vi "uTTA_CheckForErrors.vi"(8 "error in":errorcluster, 11 "Received":string) -> (0 "error out":errorcluster)   [LabVIEW 2021]
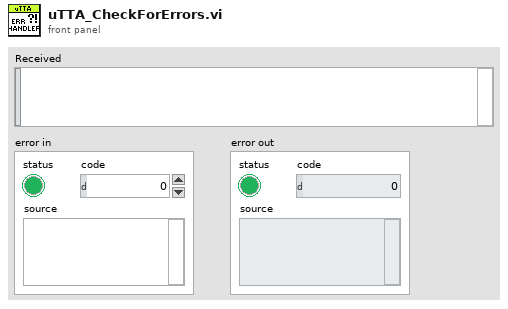
[diagram p1: front panel]
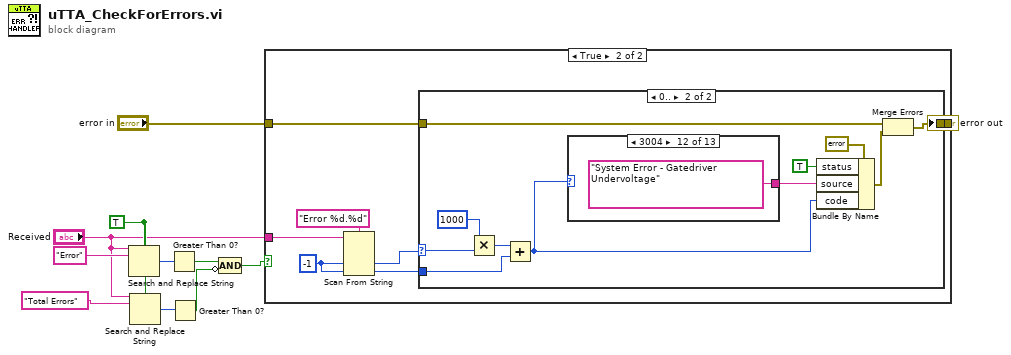
[diagram p0: block diagram]
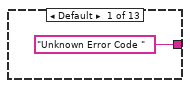
[diagram p4: hidden frame]
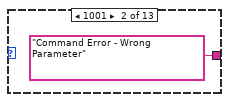
[diagram p5: hidden frame]
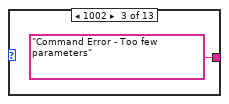
[diagram p6: hidden frame]
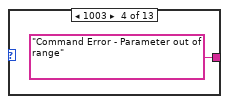
[diagram p7: hidden frame]
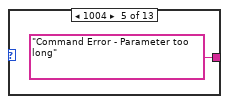
[diagram p8: hidden frame]
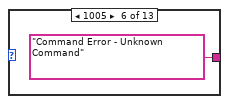
[diagram p9: hidden frame]
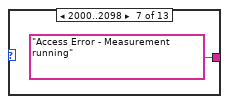
[diagram p10: hidden frame]
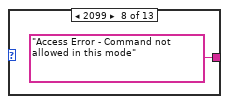
[diagram p11: hidden frame]
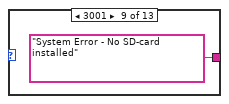
[diagram p12: hidden frame]
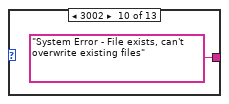
[diagram p13: hidden frame]
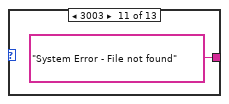
[diagram p14: hidden frame]
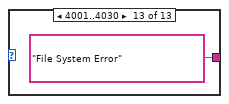
[diagram p15: hidden frame]
diagram:
  w8 = TRUE ("ignore case? (F)")
  n1 = Search and Replace String(case sensitive?=w8, input string="Received", search string="Error" ("format string")) -> (number of replacements=w4:i32)  [unwired: 5 in, 3 out]
  n2 = Search and Replace String(case sensitive?=w8, input string="Received", search string="Total Errors" ("format string")) -> (number of replacements=w5:i32)  [unwired: 5 in, 3 out]
  n3 = Greater Than 0?(x=w4) -> (x > 0?=w3:bool)
  n4 = Greater Than 0?(x=w5) -> (x > 0?=w2:bool)
  n5 = Compound Arithmetic op=AND(w3, invert w2) -> (w1:bool)
  n6 = case shown="True" w1 {
    tunnel: [w12 w19] -> w11
    tunnel: "error in" -> [w12 w18]
    tunnel: "Received" -> [_ w13]
    frame False {
    }
    frame True {
      w16 = -1 ("default value 1")
      n7 = Scan From String(format string="Error %d.%d", input string=w13, default 1=w16, default 2=w16) -> (output 1=w15:i32, output 2=w14:i32)  [unwired: 2 in, 3 out]
      n8 = case shown="0.." w15 {
        selector: w15 -> [_ w23]
        tunnel: w18 -> [w20 w31]
        tunnel: [w20 w30] -> w19
        tunnel: w14 -> [_ w25]
        frame Default {
        }
        frame 0.. {
          n9 = Multiply(x=1000, y=w23) -> (x*y=w22:i32)
          n10 = Add(x=w22, y=w25) -> (x+y=w21:i32)
          n11 = case shown="3004" w21 {
            tunnel: ["Unknown Error Code " ("source") "Command Error - Wrong Parameter" ("source") "Command Error - Too few parameters" ("source") "Command Error - Parameter out of range" ("source") "Command Error - Parameter too long" ("source") "Command Error - Unknown Command" ("source") "Access Error - Measurement running" ("source") "Access Error - Command not allowed in this mode" ("source") "System Error - No SD-card installed" ("source") "System Error - File exists, can't overwrite existing files" ("source") "System Error - File not found" ("source") "System Error - Gatedriver Undervoltage" ("source") "File System Error" ("source")] -> w26
            frame Default {
            }
            frame 1001 {
            }
            frame 1002 {
            }
            frame 1003 {
            }
            frame 1004 {
            }
            frame 1005 {
            }
            frame 2000..2098 {
            }
            frame 2099 {
            }
            frame 3001 {
            }
            frame 3002 {
            }
            frame 3003 {
            }
            frame 3004 {
            }
            frame 4001..4030 {
            }
          }
          n12 = Bundle By Name(cluster=errorcluster {"status"=FALSE, "code"=0, "source"=""} ("error in"), "status"=TRUE, "source"=w26, "code"=w21) -> (w28:errorcluster)
          n13 = Merge Errors(w31, w28) -> (w30:errorcluster)
        }
      }
    }
  }
  "error out" <- w11
